vi "HXG2_ProgammerParseData.vi"(7 "Parse Ctrl":enum16{"Write", "Pass"}(ring), 8 "error in (no error)":errorcluster, 9 "Table Data In":string[][](table)) -> (0 "error out":errorcluster, 3 "Step Array Out":T1[](array[typedef]))   [LabVIEW 2012]
doc: "Parse strings from table control for use in the array of the programmer\nAll Stability times are multiplied by 60 to pass info to programmer in seconds"
uses:
  Modules/Programmer/Data Types/Programmer Step.ctl
  Modules/Programmer/Data Types/Programmer Step References.ctl
panel:
  out "size(s) 2":i32
  out "element":i32
  out "Array":string[](array[string])
  out "size(s)":i32[](array[numeric])
  out "subarray":string[][](array[string])
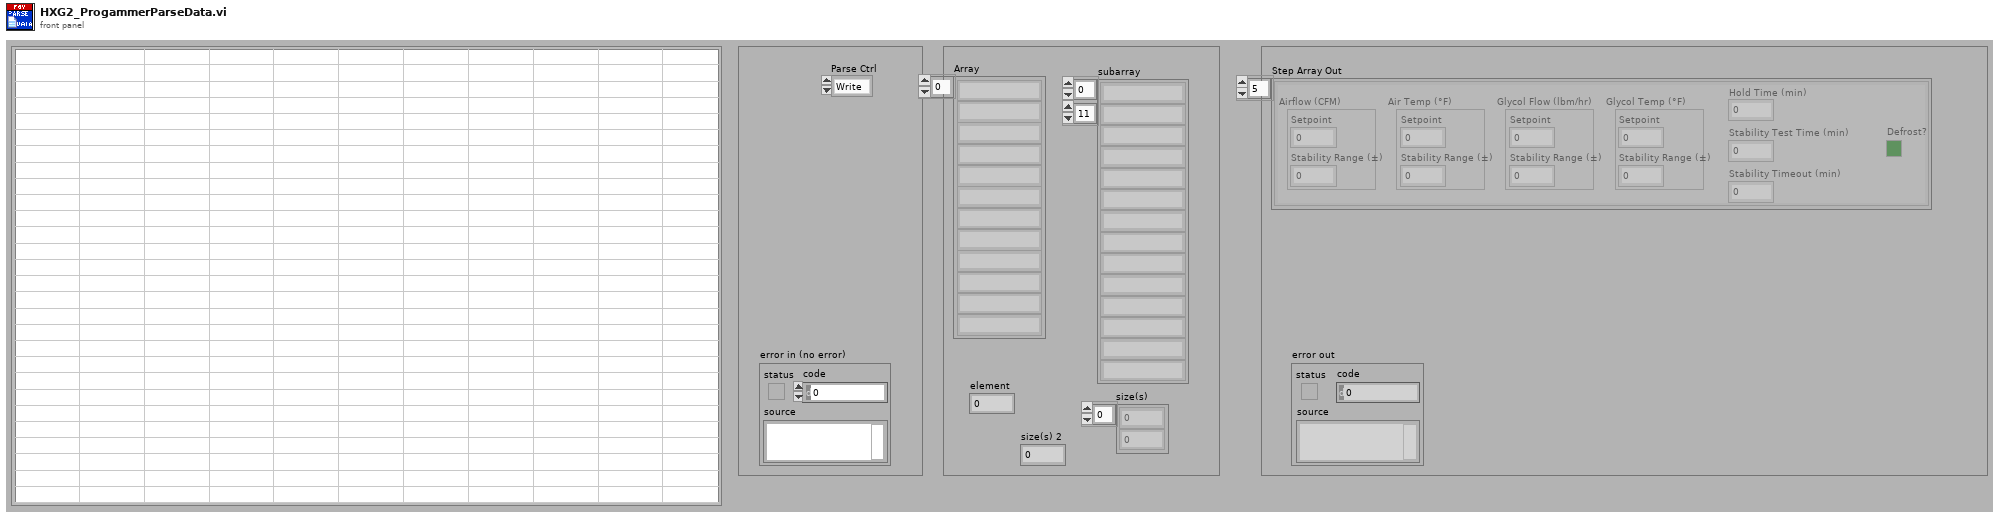
[diagram p1: front panel]
types:
  T1 = typedef "Programmer Step.ctl" = cluster{"Airflow (CFM)":T2, "Air Temp (°F)":T2, "Glycol Flow (lbm/hr)":T2, "Glycol Temp (°F)":T2, "Hold Time (min)":dbl, "Stability Test Time (min)":dbl, "Stability Timeout (min)":dbl, "Defrost?":bool}
  T2 = typedef "Programmer Step References.ctl" = cluster{"Setpoint":dbl, "Stability Range (±)":dbl}
  T3 = cluster{"[0]":dbl, "[1]":dbl, "[2]":dbl, "[3]":dbl, "[4]":dbl, "[5]":dbl, "[6]":dbl, "[7]":dbl, "[8]":dbl, "[9]":dbl, "[10]":dbl, "[11]":dbl}
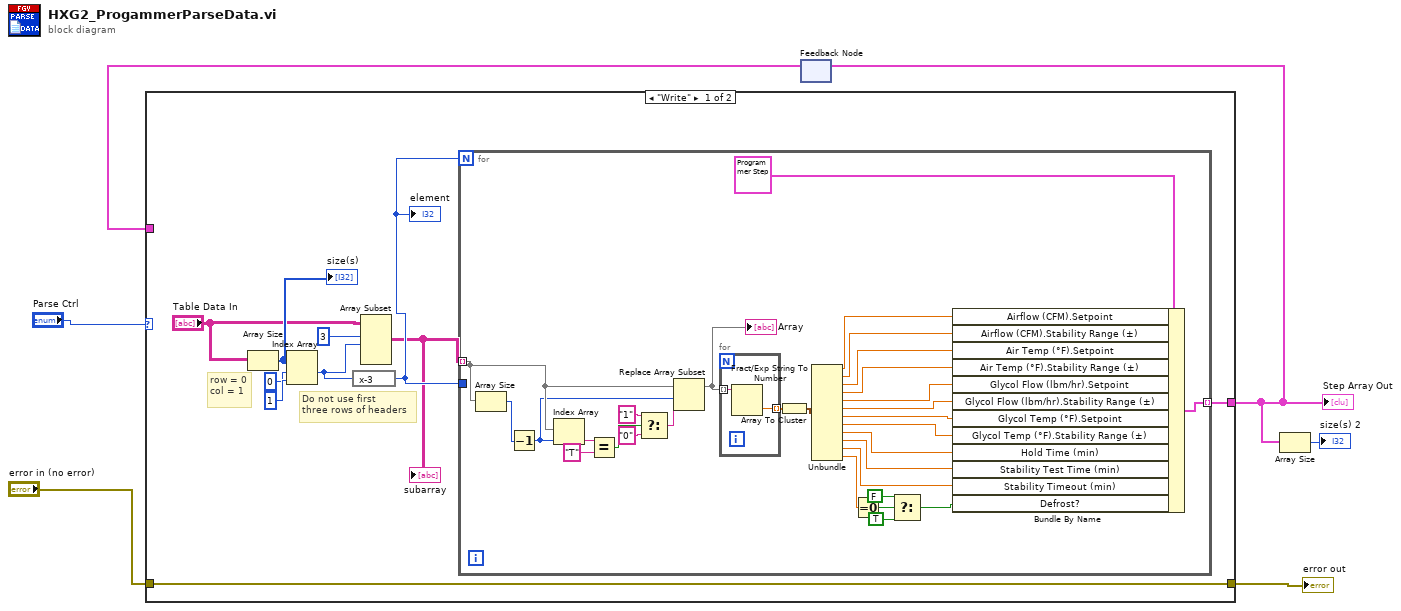
[diagram p0: block diagram]
diagram:
  n1 = feedback #1() -> (w6:T1[])  [unwired: 1 in]
  n2 = case shown="\"Write\"" "Parse Ctrl" {
    tunnel: [w12 w50] -> w2
    tunnel: w6 -> [_ w50]
    tunnel: "error in (no error)" -> [w10 w49]
    tunnel: [w10 w49] -> w3
    frame "Write" {
      # "Do not use first \nthree rows of headers"
      # "row = 0\ncol = 1"
      n3 = Array Size(array="Table Data In") -> (size(s)=w14:i32[])
      "size(s)" <- w14
      n4 = Index Array(array=w14, index #1=0 ("index"), index #2=1 ("index")) -> (element #1=w8:i32)  [unwired: 1 out]
      n5 = expression code="x-3"(w8) -> (w11:i32)
      "element" <- w11
      n6 = Array Subset(array="Table Data In", index (row)=3, length (row)=w8) -> (w7:string[][])  [unwired: 2 in]
      "subarray" <- w7
      n7 = for {
        N: w11 -> [_]
        tunnel: w7 -> [w26] mode=indexing
        tunnel: [w46] -> w12 mode=indexing
        tunnel: w11 -> [_]
        n8 = Array Size(array=w26) -> (size(s)=w25:i32)
        n9 = Decrement(x=w25) -> (x-1=w17:i32)
        n10 = Index Array(array=w26, index=w17) -> (element=w24:string)
        n11 = Equal?(x=w24, y="T") -> (x = y?=w22:bool)
        n12 = Select(t="1" ("y"), s=w22, f="0" ("y")) -> (s? t:f=w19:string)
        n13 = Replace Array Subset(array=w26, new element=w19, index=w17) -> (w18:string[])
        "Array" <- w18
        n14 = for {
          tunnel: w18 -> [w48] mode=indexing
          tunnel: [w47] -> w44 mode=indexing
          n15 = Fract/Exp String To Number(string=w48) -> (number=w47:dbl)  [unwired: 3 in, 1 out]
        }
        n16 = Array To Cluster(array=w44) -> (cluster=w43:T3)
        n17 = Unbundle(w43) -> ("[0]"=w42:dbl, "[1]"=w41:dbl, "[2]"=w40:dbl, "[3]"=w39:dbl, "[4]"=w38:dbl, "[5]"=w37:dbl, "[6]"=w36:dbl, "[7]"=w35:dbl, "[8]"=w34:dbl, "[9]"=w33:dbl, "[10]"=w32:dbl, "[11]"=w31:dbl)
        n18 = Equal To 0?(x=w31) -> (x = 0?=w30:bool)
        n19 = Select(t=FALSE, s=w30, f=TRUE) -> (s? t:f=w27:bool)
        n20 = Bundle By Name(cluster=T1 {"Airflow (CFM)"={"Setpoint"=0.0, "Stability Range (±)"=0.0}, "Air Temp (°F)"={"Setpoint"=0.0, "Stability Range (±)"=0.0}, "Glycol Flow (lbm/hr)"={"Setpoint"=0.0, "Stability Range (±)"=0.0}, "Glycol Temp (°F)"={"Setpoint"=0.0, "Stability Range (±)"=0.0}, "Hold Time (min)"=0.0, "Stability Test Time (min)"=0.0, "Stability Timeout (min)"=0.0, "Defrost?"=FALSE} ("Programmer Step"), "Airflow (CFM).Setpoint"=w42, "Airflow (CFM).Stability Range (±)"=w41, "Air Temp (°F).Setpoint"=w40, "Air Temp (°F).Stability Range (±)"=w39, "Glycol Flow (lbm/hr).Setpoint"=w38, "Glycol Flow (lbm/hr).Stability Range (±)"=w37, "Glycol Temp (°F).Setpoint"=w36, "Glycol Temp (°F).Stability Range (±)"=w35, "Hold Time (min)"=w34, "Stability Test Time (min)"=w33, "Stability Timeout (min)"=w32, "Defrost?"=w27) -> (w46:T1)
      }
    }
    frame "Pass", Default {
    }
  }
  "error out" <- w3
  "Step Array Out" <- w2
  n21 = feedback-in #1(w2) -> ()
  n22 = Array Size(array=w2) -> (size(s)=→"size(s) 2":i32)
